vi "ShowSoftPanel.vi"(8 "error in (no error)":errorcluster, 9 "Floating":bool=TRUE, 10 "Ancestor":string, 11 "Driver in":refnum<class "ViPER.lvclass">) -> (0 "error out":errorcluster, 2 "vi reference":refnum<vi>, 3 "Driver out":refnum<class "ViPER.lvclass">)   [LabVIEW 2022 SP3, in "ViPER.lvlib" / "ViPER.lvclass"]
doc: "### BSD License (http://www.opensource.org/licenses/bsd-license.php) Begin ###\n\nCopyright (c) 2018 Kurt Friday www.medulla.net\n\nAll rights reserved.\n\nRedistribution and use in source and binary forms, with or without\nmodification, are permitted provided that the following conditions are met:\n\n * Redistributions of source code must retain the above copyright\n notice, this list of conditions and the following disclaimer.\n\n * Redistributions in binary form must reproduce the above copyright\n notice, this list of conditions and the following disclaimer in the\n documentation and/or other materials provided with the distribution.\n\n * Neither the name of the <organization> nor the\n names of its contributors may be used to endorse or promote products\n derived from this software without specific prior written permission.\n\nTHIS SOFTWARE IS PROVIDED BY THE COPYRIGHT HOLDERS AND CONTRIBUTORS \"AS IS\" AND\nANY EXPRESS OR IMPLIED WARRANTIES, INCLUDING, BUT NOT LIMITED TO, THE IMPLIED\nWARRANTIES OF MERCHANTABILITY AND FITNESS FOR A PARTICULAR PURPOSE ARE\nDISCLAIMED. IN NO EVENT SHALL <COPYRIGHT HOLDER> BE LIABLE FOR ANY\nDIRECT, INDIRECT, INCIDENTAL, SPECIAL, EXEMPLARY, OR CONSEQUENTIAL DAMAGES\n(INCLUDING, BUT NOT LIMITED TO, PROCUREMENT OF SUBSTITUTE GOODS OR SERVICES;\nLOSS OF USE, DATA, OR PROFITS; OR BUSINESS INTERRUPTION) HOWEVER CAUSED AND\nON ANY THEORY OF LIABILITY, WHETHER IN CONTRACT, STRICT LIABILITY, OR TORT\n(INCLUDING NEGLIGENCE OR OTHERWISE) ARISING IN ANY WAY OUT OF THE USE OF THIS\nSOFTWARE, EVEN IF ADVISED OF THE POSSIBILITY OF SUCH DAMAGE."
uses:
  ViPER.lvclass
panel:
  # "### BSD License (http://www.opensource.org/licenses/bsd-license.php) Begin ###\n\nCopyright (c) 2018  Kurt Friday www.medulla.net\n\nAll rights reserved.\n\nRedistribution and use in source and binary forms, with or without\nmodification, are permitted provided that the following conditions are met:\n\n    * Redistributions of source code must retain the above copyright\n      notice, this list of conditions and the following disclaimer.\n\n    * Redistributions in binary form must reproduce the above copyright\n      notice, this list of conditions and the following disclaimer in the\n      documentation and/or other materials provided with the distribution.\n\n    * Neither the name of the <organization> nor the\n      names of its contributors may be used to endorse or promote products\n      derived from this software without specific prior written permission.\n\nTHIS SOFTWARE IS PROVIDED BY THE COPYRIGHT HOLDERS AND CONTRIBUTORS \"AS IS\" AND\nANY EXPRESS OR IMPLIED WARRANTIES, INCLUDING, BUT NOT LIMITED TO, THE IMPLIED\nWARRANTIES OF MERCHANTABILITY AND FITNESS FOR A PARTICULAR PURPOSE ARE\nDISCLAIMED. IN NO EVENT SHALL <COPYRIGHT HOLDER> BE LIABLE FOR ANY\nDIRECT, INDIRECT, INCIDENTAL, SPECIAL, EXEMPLARY, OR CONSEQUENTIAL DAMAGES\n(INCLUDING, BUT NOT LIMITED TO, PROCUREMENT OF SUBSTITUTE GOODS OR SERVICES;\nLOSS OF USE, DATA, OR PROFITS; OR BUSINESS INTERRUPTION) HOWEVER CAUSED AND\nON ANY THEORY OF LIABILITY, WHETHER IN CONTRACT, STRICT LIABILITY, OR TORT\n(INCLUDING NEGLIGENCE OR OTHERWISE) ARISING IN ANY WAY OUT OF THE USE OF THIS\nSOFTWARE, EVEN IF ADVISED OF THE POSSIBILITY OF SUCH DAMAGE."
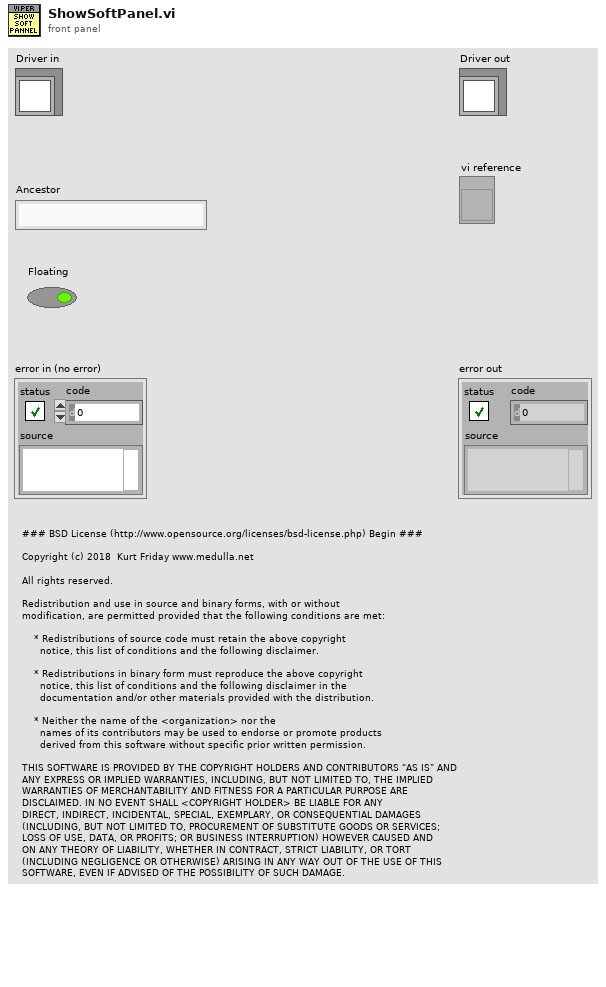
[diagram p1: front panel]
types:
  T1 = enum32{"Invalid", "Standard", "Closed", "Hidden", "Minimized", "Maximized"}
  T2 = typedef "ViPER.lvlib/ViPER.lvclass/Details.ctl" = cluster{"Name":string, "Class":string}
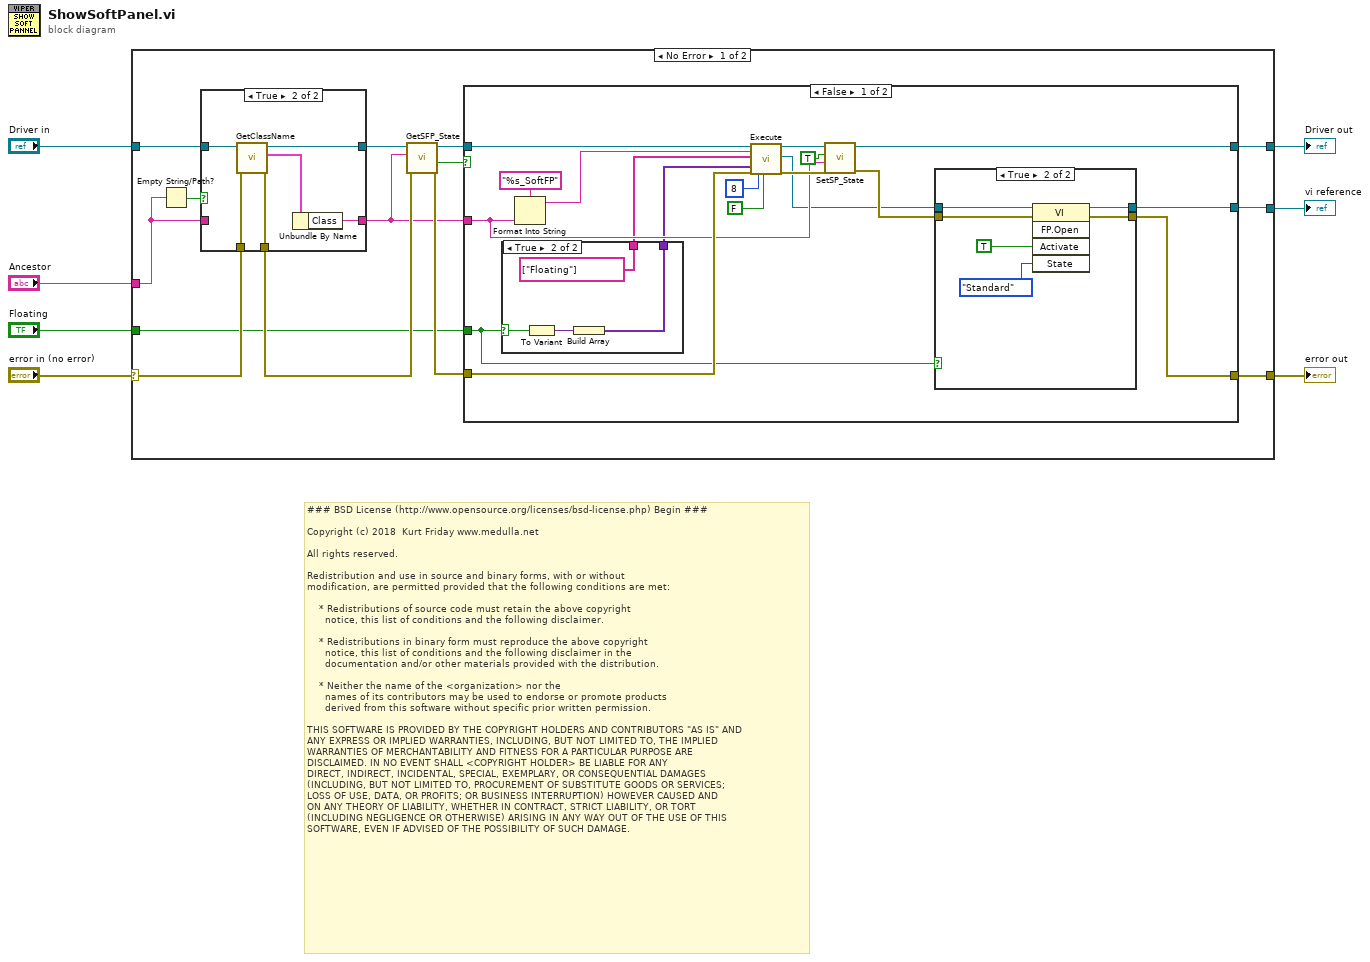
[diagram p0: block diagram]
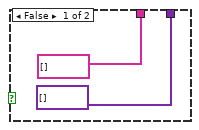
[diagram p4: hidden frame]
diagram:
  # "### BSD License (http://www.opensource.org/licenses/bsd-license.php) Begin ###\n\nCopyright (c) 2018  Kurt Friday www.medulla.net\n\nAll rights reserved.\n\nRedistribution and use in source and binary forms, with or without\nmodification, are permitted provided that the following conditions are met:\n\n    * Redistributions of source code must retain the above copyright\n      notice, this list of conditions and the following disclaimer.\n\n    * Redistributions in binary form must reproduce the above copyright\n      notice, this list of conditions and the following disclaimer in the\n      documentation and/or other materials provided with the distribution.\n\n    * Neither the name of the <organization> nor the\n      names of its contributors may be used to endorse or promote products\n      derived from this software without specific prior written permission.\n\nTHIS SOFTWARE IS PROVIDED BY THE COPYRIGHT HOLDERS AND CONTRIBUTORS \"AS IS\" AND\nANY EXPRESS OR IMPLIED WARRANTIES, INCLUDING, BUT NOT LIMITED TO, THE IMPLIED\nWARRANTIES OF MERCHANTABILITY AND FITNESS FOR A PARTICULAR PURPOSE ARE\nDISCLAIMED. IN NO EVENT SHALL <COPYRIGHT HOLDER> BE LIABLE FOR ANY\nDIRECT, INDIRECT, INCIDENTAL, SPECIAL, EXEMPLARY, OR CONSEQUENTIAL DAMAGES\n(INCLUDING, BUT NOT LIMITED TO, PROCUREMENT OF SUBSTITUTE GOODS OR SERVICES;\nLOSS OF USE, DATA, OR PROFITS; OR BUSINESS INTERRUPTION) HOWEVER CAUSED AND\nON ANY THEORY OF LIABILITY, WHETHER IN CONTRACT, STRICT LIABILITY, OR TORT\n(INCLUDING NEGLIGENCE OR OTHERWISE) ARISING IN ANY WAY OUT OF THE USE OF THIS\nSOFTWARE, EVEN IF ADVISED OF THE POSSIBILITY OF SUCH DAMAGE."
  n1 = case shown="No Error" "error in (no error)" {
    selector: "error in (no error)" -> [w14 w66]
    tunnel: [w18 w66] -> w6
    tunnel: "Driver in" -> [w16 w65]
    tunnel: [w17 w65] -> w4
    tunnel: "Ancestor" -> [w11 _]
    tunnel: [w9 _] -> w2
    tunnel: "Floating" -> [w8 _]
    frame No Error {
      n2 = Empty String/Path?(string/path=w11) -> (empty?=w12:bool)
      n3 = case shown="True" w12 {
        tunnel: w14 -> [w23 w30]
        tunnel: [w23 w29] -> w13
        tunnel: w16 -> [w24 w28]
        tunnel: [w24 w27] -> w15
        tunnel: w11 -> [w22 _]
        tunnel: [w22 w25] -> w10
        frame False {
        }
        frame True {
          n4 = call "GetClassName.vi"("error in (no error)"=w30, "reference in"=w28) -> ("error out"=w29:errorcluster, "Details"=w26:T2, "reference out"=w27:refnum<class "ViPER.lvclass">)  [unwired: 7 in]
          n5 = Unbundle By Name(w26) -> ("Class"=w25:string)
        }
      }
      n6 = call-dynamic "GetSFP_State.vi"("error in (no error)"=w13, "Ancestor"=w10, "reference in"=w15) -> ("error out"=w21:errorcluster, "SP_open"=w19:bool, "reference out"=w20:refnum<class "ViPER.lvclass">)  [unwired: 6 in]
      n7 = case shown="False" w19 {
        tunnel: w21 -> [w48 w63]
        tunnel: w20 -> [w47 w64]
        tunnel: [w34 w63] -> w18
        tunnel: [w43 w64] -> w17
        tunnel: w10 -> [w38 _]
        tunnel: [w32 _] -> w9
        tunnel: w8 -> [w31 _]
        frame False {
          n8 = case shown="True" w31 {
            selector: w31 -> [_ w59]
            tunnel: [string[] [] string[] ["Floating"]] -> w37
            tunnel: [variant[] [] w60] -> w36
            frame False {
            }
            frame True {
              n9 = To Variant(anything=w59) -> (Variant=w61:variant)
              n10 = Build Array(w61) -> (w60:variant[])
            }
          }
          n11 = Format Into String(format string="%s_SoftFP" ("method"), w38) -> (resulting string=w39:string)  [unwired: 2 in, 1 out]
          n12 = call-dynamic "Execute.vi"("reference in"=w47, "cmd"=w39, "controls"=w37, "control data"=w36, "error in (no error)"=w48, "options"=8, "wait until done (T)"=FALSE) -> ("reference out"=w45:refnum<class "ViPER.lvclass">, "vi reference"=w33:refnum<vi>, "error out"=w46:errorcluster)  [unwired: 8 in, 2 out]
          n13 = call "SetSP_State.vi"("error in (no error)"=w46, "Ancestor"=w38, "SP Open"=TRUE, "reference in"=w45) -> ("error out"=w35:errorcluster, "reference out"=w43:refnum<class "ViPER.lvclass">)  [unwired: 6 in]
          n14 = case shown="True" w31 {
            tunnel: w35 -> [w50 w54]
            tunnel: [w50 w53] -> w34
            tunnel: w33 -> [w49 w52]
            tunnel: [w49 w51] -> w32
            frame False {
            }
            frame True {
              n15 = invoke class="VI" method="FP.Open"(reference=w52, error in=w54, "Activate"=TRUE ("Activate?"), "State"=T1."Standard") -> (reference out=w51:refnum<vi>, error out=w53:errorcluster)  [unwired: 1 in, 3 out]
            }
          }
        }
        frame True {
        }
      }
    }
    frame Error {
    }
  }
  "error out" <- w6
  "Driver out" <- w4
  "vi reference" <- w2
